vi "Value with SI prefix To Value with SI prefix.vi"(7 "Output Prefix":T1, 8 "error in":errorcluster, 10 "Unit In":T2, 11 "Scaled Value":dbl format="%#.6f") -> (0 "error out":errorcluster, 2 "Unit (with prefix)":T2, 3 "Value":dbl format="%#.6f")   [LabVIEW 2013, in "Mercury iXX.lvlib"]
doc: "This VI converts a numeric input with SI prefix into a numeric with a user-selectable SI prefix."
uses:
  <instrlib>/Mercury iXX/Mercury iXX.lvlib
  <instrlib>/Mercury iXX/Public/Controls/Unit String.ctl
  <instrlib>/Mercury iXX/Public/Controls/SI Prefix.ctl
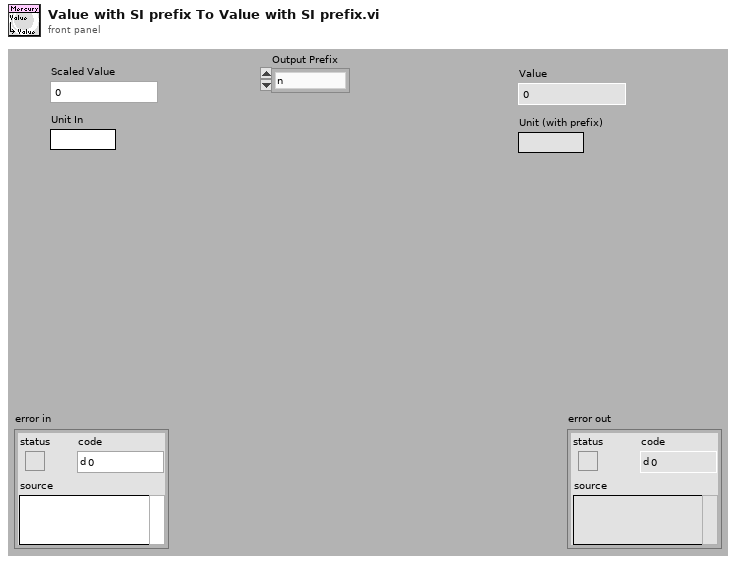
[diagram p1: front panel]
types:
  T1 = typedef "Mercury iXX.lvlib/SI Prefix.ctl" = enum16{"n", "µ", "m", "No Prefix", "k", "M", "G"}
  T2 = typedef "Mercury iXX.lvlib/Unit String.ctl" = string
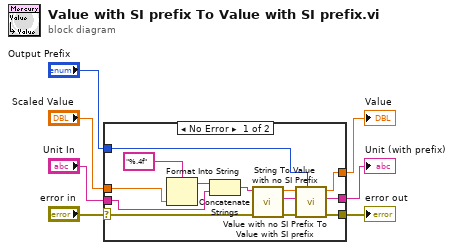
[diagram p0: block diagram]
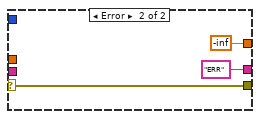
[diagram p2: hidden frame]
diagram:
  n1 = case shown="No Error" "error in" {
    selector: "error in" -> [w18 w23]
    tunnel: [w17 w23] -> w6
    tunnel: [w16 -inf] -> w5
    tunnel: [w15 "ERR" ("Unit-")] -> w4
    tunnel: "Scaled Value" -> [w20 _]
    tunnel: "Unit In" -> [w19 _]
    tunnel: "Output Prefix" -> [w14 _]
    frame No Error {
      n2 = Format Into String(format string="%.4f", w20) -> (resulting string=w9:string)  [unwired: 2 in, 1 out]
      n3 = Concatenate Strings(w9, w19) -> (w8:string)
      n4 = call <instrlib>:"String To Value with no SI Prefix.vi"("error in"=w18, "Response"=w8) -> ("error out"=w11:errorcluster, "Unit"=w13:T2, "Scaled Value"=w12:dbl)  [unwired: 7 out]
      n5 = call <instrlib>:"Value with no SI Prefix To Value with SI prefix.vi"("Output Prefix"=w14, "error in"=w11, "Unit In"=w13, "Scaled Value"=w12) -> ("error out"=w17:errorcluster, "Unit (with prefix)"=w15:T2, "Value"=w16:dbl)  [unwired: 5 out]
    }
    frame Error {
    }
  }
  "error out" <- w6
  "Value" <- w5
  "Unit (with prefix)" <- w4
